vi "From STFT Spectrogram Demo.vi"() -> ()   [LabVIEW 2022 SP3]
doc: "This example demonstrates how to use the STFT Spectrograms VI to analyze the Time-Frequency spectrogram.\n\nInstructions:\n1) Run the VI.\n\n2) Change the <b>time-freq sampling info</b> to see the effect of the different <b>time steps</b> or <b>frequency bins</b> on the spectrogram.\n\n3) Change the window <b>type</b> or <b>length</b> to see the effect of different windows on the spectrogram."
uses:
  <vilib>/gmath/NI_Gmath.lvlib
panel:
  in  "window info":cluster{"type":u32, "length":i32}={"type"=1, "length"=64} {"type" items=["Rectangle"=0, "Hanning"=1, "Hamming"=2, "Blackman-Harris"=3, "Exact Blackman"=4, "Blackman"=5, "Flat Top"=6, "4 Term B-Harris "=7, "7 Term B-Harris"=8, "Low Sidelobe"=9, "Blackman Nuttall"=11, "Triangle"=30, "Gaussian"=62]}
  in  "sampling rate (Hz)":i32=100000 min=1000 step=1
  out "Signal":dynamicdata(graph)
  out "STFT Spectrogram":dbl[][](graph)
  in  "stop":bool
  in  "time-freq sampling info":cluster{"time steps":i32, "frequency bins":i32}={"time steps"=4, "frequency bins"=32}
  # "Select Help>>Show Context Help and move the cursor over the VI icon to display help for this VI."
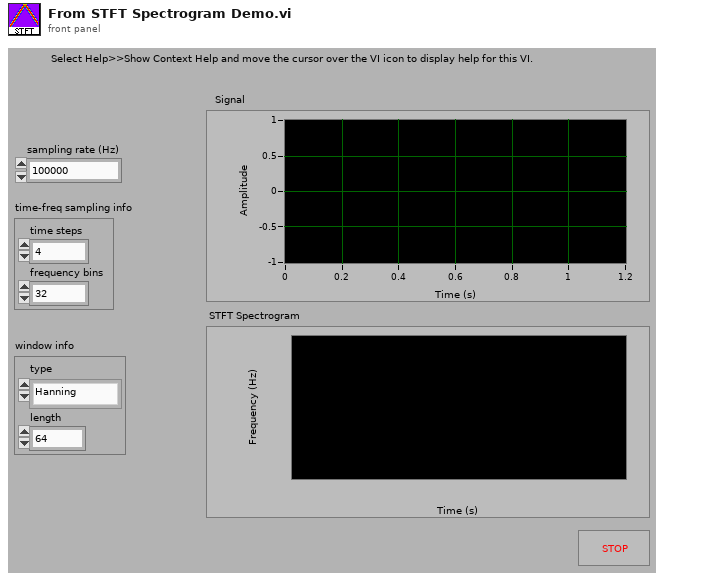
[diagram p1: front panel]
types:
  T1 = enum16{"fire", "rainbow", "grey", "inverse grey", "ice", "original"}
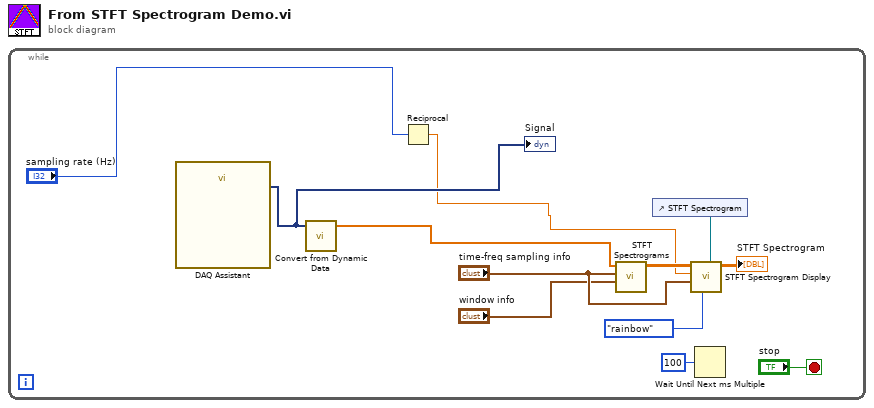
[diagram p0: block diagram]
diagram:
  n1 = while {
    stop <- "stop" stop-if-true
    n2 = call "DAQ Assistant"() -> ("data"=w3:dynamicdata)  [unwired: 5 in, 14 out]
    "Signal" <- w3
    n3 = call "Convert from Dynamic Data"("Dynamic Data Type"=w3) -> ("Array"=w2:dbl[])  [unwired: 3 out]
    n4 = Reciprocal(x="sampling rate (Hz)") -> (1/x=w1:dbl)
    n5 = call <vilib>:"STFT Spectrograms.vi"("window info"="window info", "time-freq sampling info"="time-freq sampling info", "X"=w2) -> ("STFT Spectrogram {X}"=w8:dbl[][])  [unwired: 3 in, 5 out]
    n6 = control-ref of="STFT Spectrogram"() -> (w9:refnum<vi>)
    n7 = call "STFT Spectrogram Display.vi"("Intensity Graph"=w9, "map selector"=T1."rainbow", "time-freq sampling info"="time-freq sampling info", "dt"=w1, "STFT Spectrogram In"=w8) -> ("STFT Spectrogram Out"=→"STFT Spectrogram":dbl[][])  [unwired: 2 in, 4 out]
    n8 = Wait Until Next ms Multiple(millisecond multiple=u32 100) -> ()  [unwired: 1 out]
  }
